vi "Enqueue Multiple Elements.vi"(6 "Priority":T2, 8 "error in (no error)":errorcluster, 11 "QDMH in":refnum<class "QDMH.lvclass">) -> (0 "error out":errorcluster, 3 "QDMH out":refnum<class "QDMH.lvclass">)   [LabVIEW 2023, in "QDMH.lvlib" / "QDMH.lvclass"]
doc: "Enqueue Fully Formed message with data array\nPriority determines if the item is enqueued at the end of the stack or the front and how the array is organized\n\nLow: Add to End\nHigh: Reverse array and add to front"
uses:
  Library/QDMH.lvclass
  Custom Controls/Enqueue Priority.ctl
  Custom Controls/Message.ctl
panel:
  in  "Messages":T1[](array[typedef])
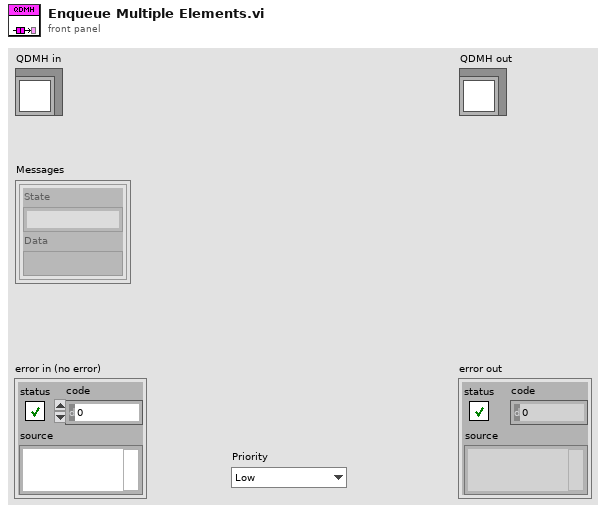
[diagram p1: front panel]
types:
  T1 = typedef "QDMH.lvlib/QDMH.lvclass/Message.ctl" = cluster{"State":string, "Data":variant}
  T2 = typedef "QDMH.lvlib/QDMH.lvclass/Enqueue Priority.ctl" = enum16{"Low", "High"}
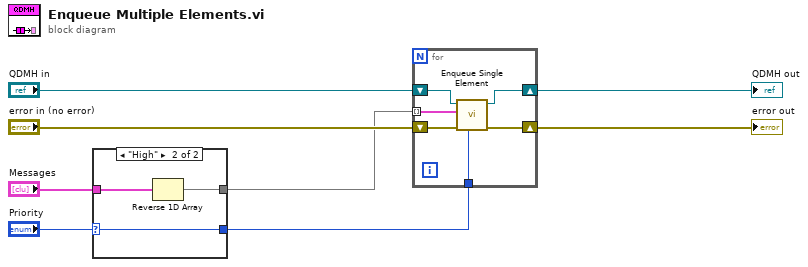
[diagram p0: block diagram]
diagram:
  n1 = case shown="\"High\"" "Priority" {
    selector: "Priority" -> [w10 w13]
    tunnel: [w10 w13] -> w3
    tunnel: "Messages" -> [w9 w12]
    tunnel: [w9 w11] -> w1
    frame "Low", Default {
    }
    frame "High" {
      n2 = Reverse 1D Array(array=w12) -> (reversed array=w11:T1[])
    }
  }
  n3 = for {
    tunnel: w3 -> [w15]
    tunnel: w1 -> [w14] mode=indexing
    shift-right: [w18] -> w7
    shift-left: "QDMH in" -> [w19]
    shift-right: [w16] -> w5
    shift-left: "error in (no error)" -> [w17]
    n4 = call "Enqueue Single Element.vi"("Priority"=w15, "error in (no error)"=w17, "Message"=w14, "QDMH in"=w19) -> ("error out"=w16:errorcluster, "QDMH out"=w18:refnum<class "QDMH.lvclass">)  [unwired: 6 in]
  }
  "error out" <- w5
  "QDMH out" <- w7
